vi "MarvinTester.vi"() -> ()   [LabVIEW 2017]
uses:
  <vilib>/Instr/_visa.llb/VISA Configure Serial Port (Instr).vi
panel:
  out "TX":string
  out "RX":string
  out "(hi.lo)":u32 format="%.0x"
  in  "GetOUTIO3":bool
  out "S2 GIO 19":bool
  out "S2 GIO 18":bool
  out "S2 GIO 17":bool
  out "S2 GIO 11":bool
  out "S2 GIO 3":bool
  out "S2 GIO 1":bool
  out "S1 GIO 19":bool
  out "S1 GIO 18":bool
  out "S1 GIO 17":bool
  out "S1 GIO 15":bool
  out "S1 GIO 11":bool
  out "S1 GIO 3":bool
  out "S1 GIO 1":bool
  in  "GetIO 2":bool
  out "S2 GIO 15 R":bool
  in  "Reset":bool
  in  "SetDefault":bool
  out "GetIO":u8[](array[numeric])
  out "Ver":string=" "
  in  "Get  ver":bool
  out "PWM Reading":u32
  out "Time Plot":i32=-1
  out "error out":errorcluster
  in  "stop":bool
  in  "Ring":u16(ring) items=["None", "Moment", "Get IO"]
  out "packet PWM":u8[](array[numeric])
  in  "Tab Control":enum32{"Page 3", "Page 4", "Page 2"}(tab)
  in  "GetIO2":bool
  out "out_io1":u32 format="%.0b"
  in  "SetDAC":bool
  in  "I_O":u32 format="%.0b"
  in  "ADC":bool
  in  "ADC num":u8=3
  out "out_io1 2":u32
  in  "DAC":u32
  out "x*y":dbl
  in  "idx":i32
  in  "TA[idx]":bool
  in  "Disconect 2":bool
  in  "110":bool
  in  "120":bool
  in  "90":bool
  in  "60":bool
  in  "100":bool
  in  "20":bool
  in  "70":bool
  in  "40":bool
  in  "30":bool
  in  "80":bool
  in  "50":bool
  in  "10":bool
  in  "25":bool
  in  "0":bool
  in  "COM Port Marvin":refnum<visa-resource-name>="COM1"
  in  "Connect Marvin":bool
  out "CommIcon Marvin":bool=TRUE
  out "String":string
  in  "K15":bool
  in  "Firmeware":bool
  in  "K16":bool
  in  "K17":bool
  in  "Power":bool
  in  "Fan":bool
  in  "VEnable":bool
  out "CurrSp Graph":cluster{"n":dbl, "T":dbl}[](graph)
  out "Frequency":dbl
  in  "Plot On":bool
  in  "Plot OFF":bool
  in  "Get":bool
  in  "Clear":bool
  in  "Plot Time":i32=70
  out "Load":dbl
  out "String 2":string
  in  "COM Port Control":refnum<visa-resource-name>="COM1"
  in  "Time":i32=-1
  out "err tx":errorcluster
  out "Write array":u8[](array[numeric]) format="%x"
  in  "Flag Stop T":bool
  out "VISA":refnum<visa-resource-name>
  out "CommIcon":bool=TRUE
  out "Read array":u8[](array[numeric]) format="%x"
  out "Cmd Id":u8
  in  "Flag Stop I":bool=TRUE
  out "Int b":i32
  in  "Flag Stop R":bool
  out "TX":bool
  out "RX":bool
  in  "Command Menu 2":u16(ring) items=["Status", "Moment", "Isc threshold", "Vin Vout", "RESET FF", "Open", "Close", "Up Time", "Interval Period", "Nm Of Retries", "On time", "Save Parameters", "Version", "Temperature"]
  out "packet":u8[](array[numeric])
  in  "Isc1":i8
  in  "Add Unit":u8
  in  "Disconect":bool
  in  "Connect":bool
  in  "Stop VI":bool
  out "status":bool
  # "Marvin Tester"
  # "[Hz]"
  # "SW Version"
  # "ver : 00.01.b"
  # "I/O"
  # "ADC"
  # "DAC"
  # "0-4"
  # "V=ADC*3.3/4096"
  # "Term1  -0\nTerm2  -1\nCurr   - 2\nEBAYFAN -3\nTempCPU -4"
  # "b0-Rly1\nb1-Rly2\nb2-Rly3\n....\nb20-Rly20\nb21-Power"
  # "[kHz]"
  # "[N.m]"
  # "[msec]"
  # "ver 0.0.1"
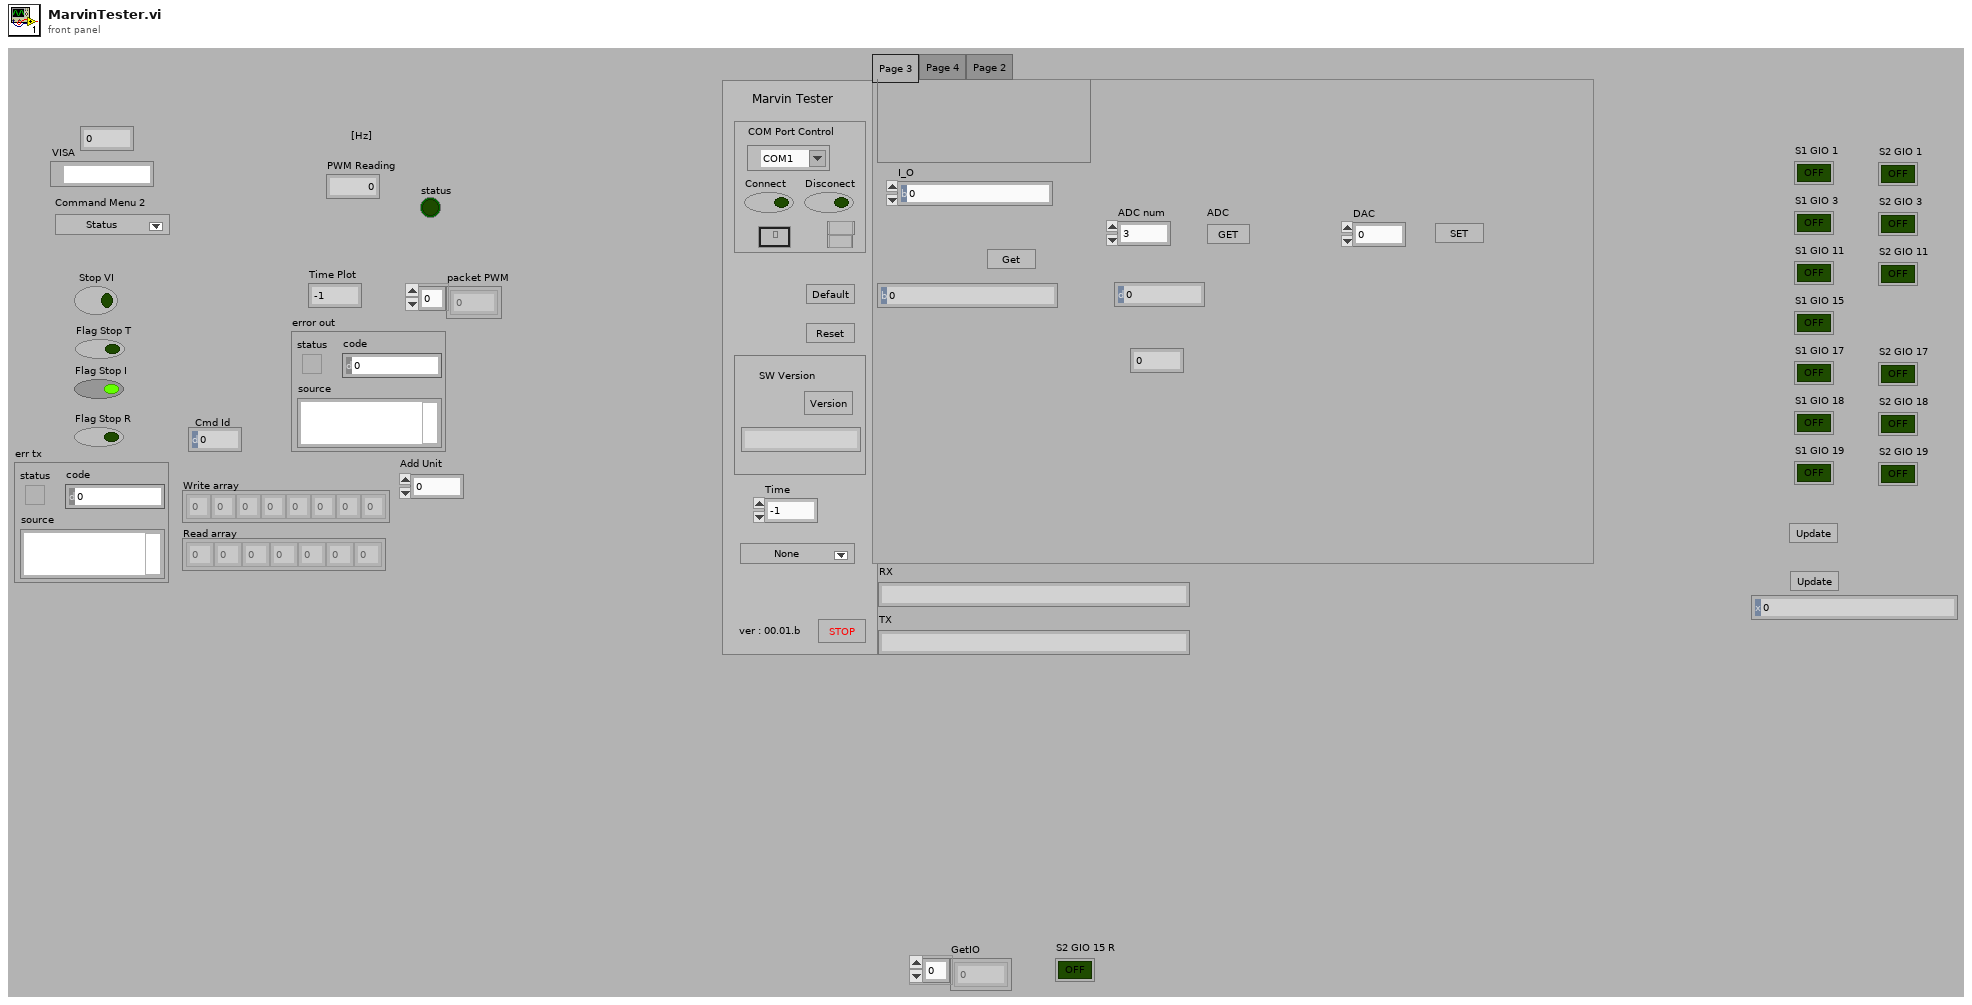
[diagram p1: front panel]
types:
  T1 = cluster{"d1":dbl, "d2":dbl, "d3":dbl, "id":u16, "d4":dbl}
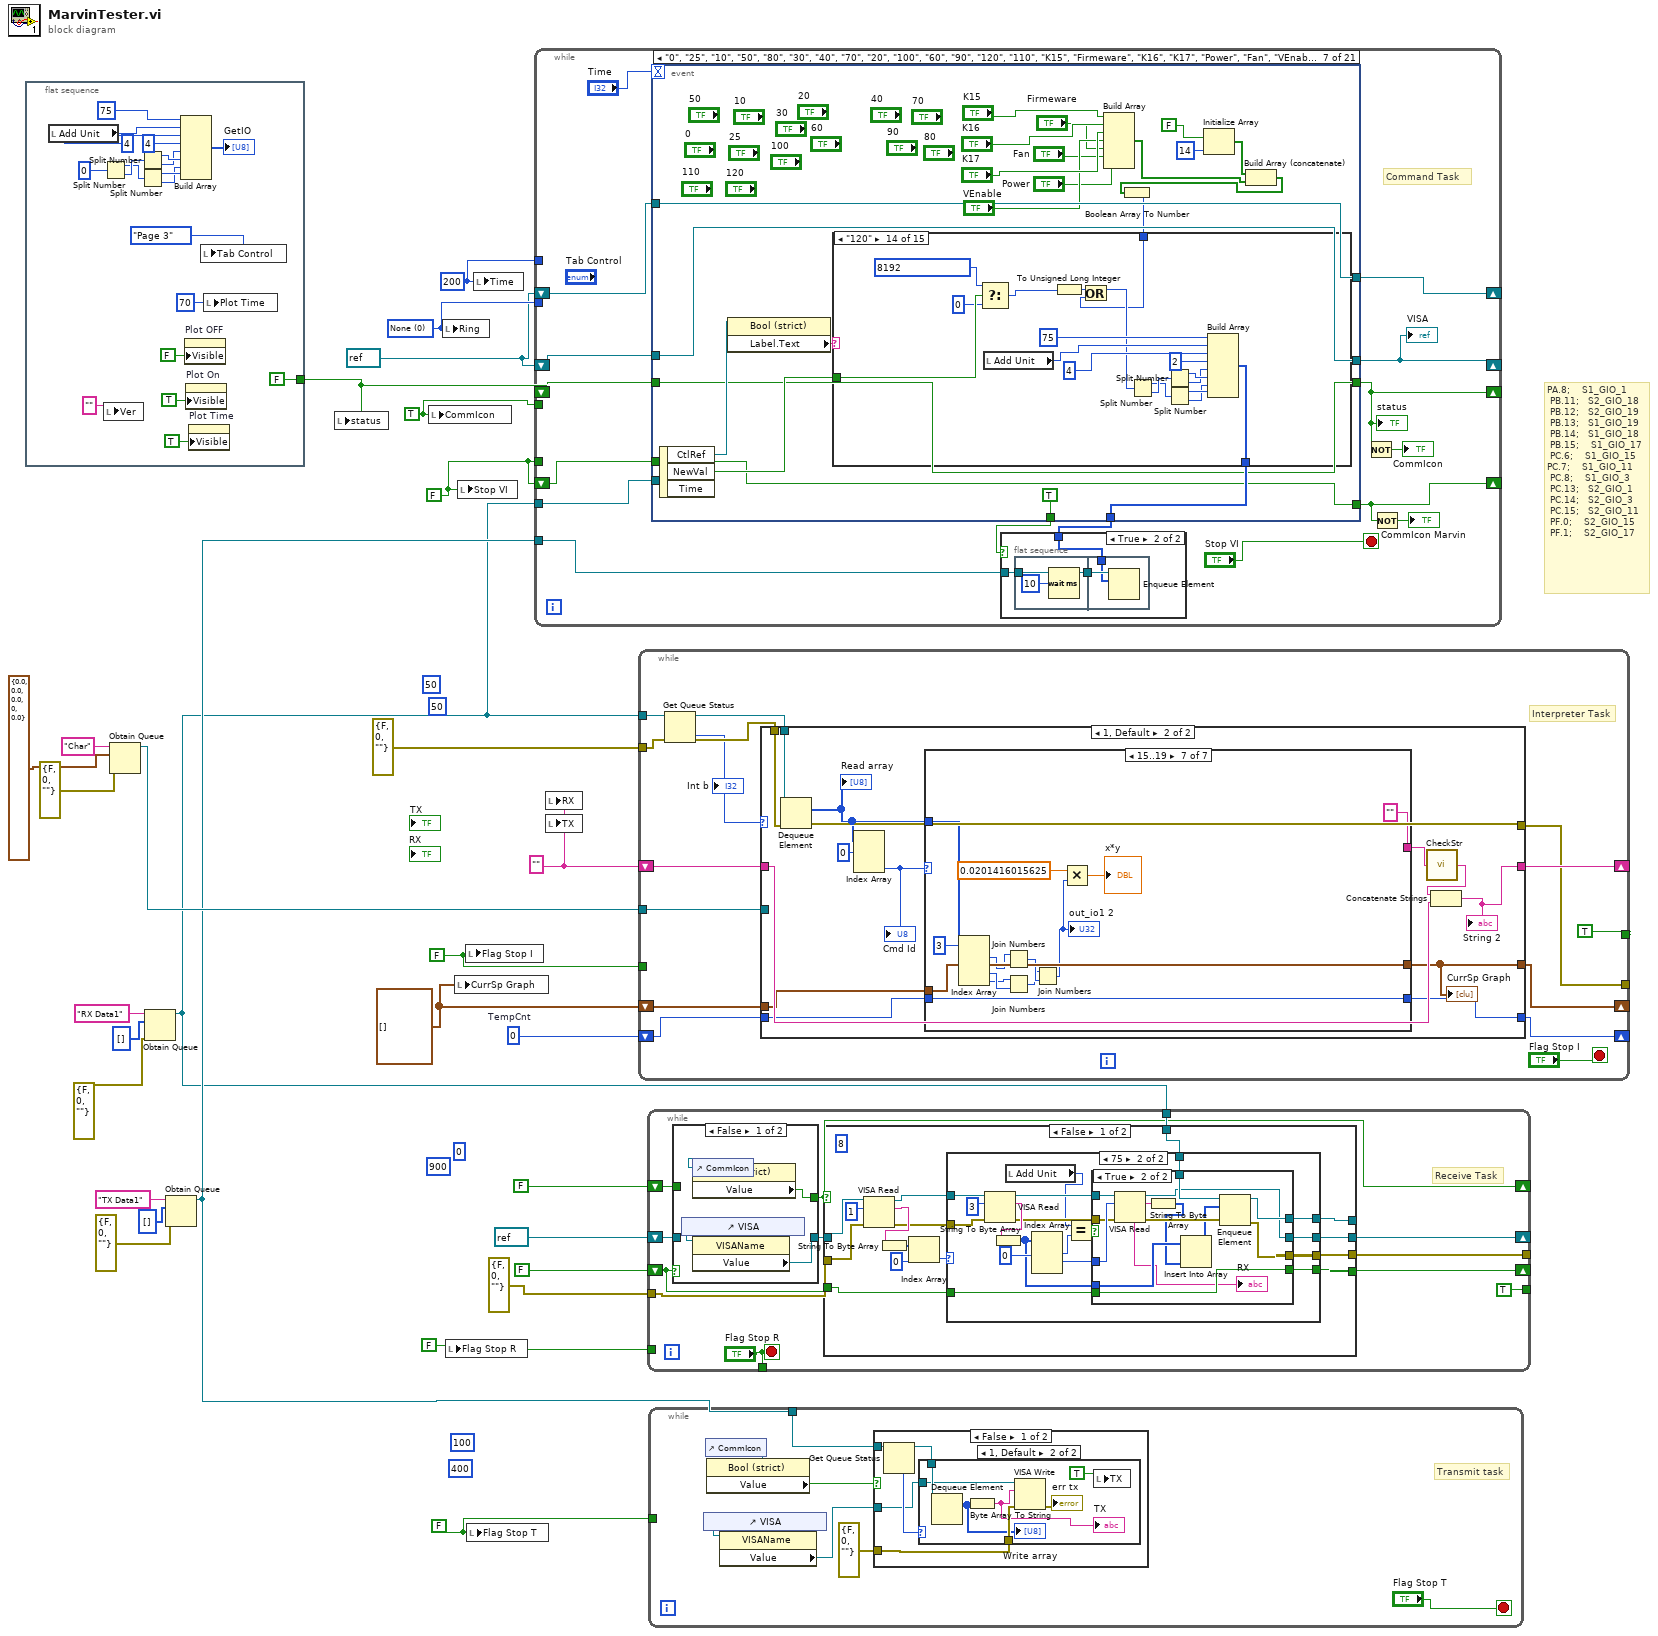
[diagram p0: block diagram]
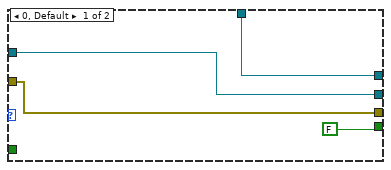
[diagram p3: hidden frame]
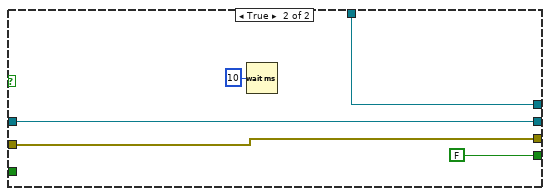
[diagram p5: hidden frame]
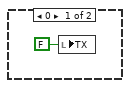
[diagram p6: hidden frame]
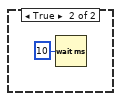
[diagram p7: hidden frame]
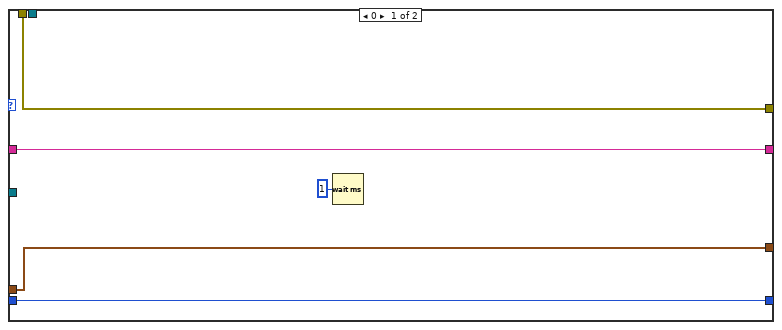
[diagram p8: hidden frame]
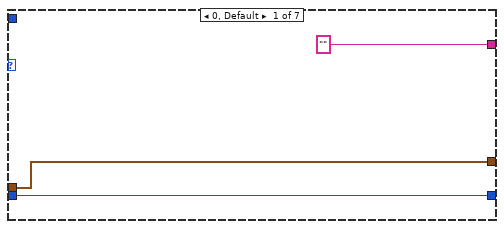
[diagram p9: hidden frame]
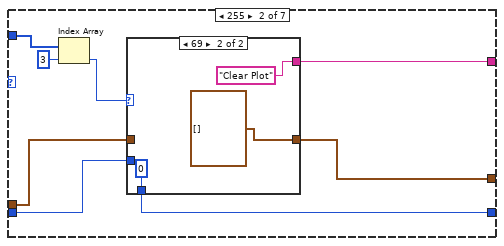
[diagram p10: hidden frame]
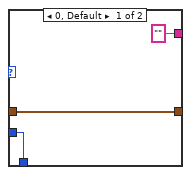
[diagram p11: hidden frame]
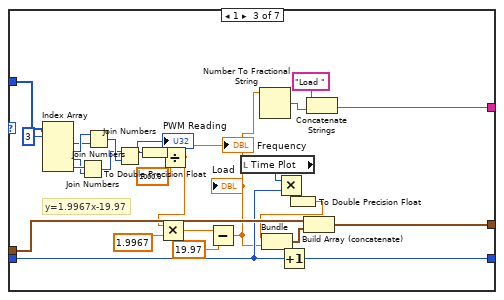
[diagram p12: hidden frame]
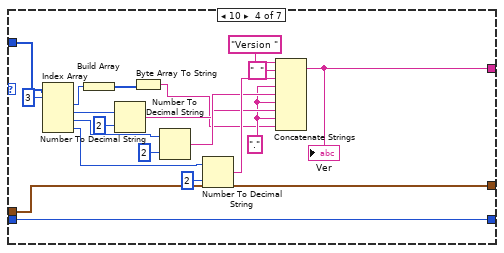
[diagram p13: hidden frame]
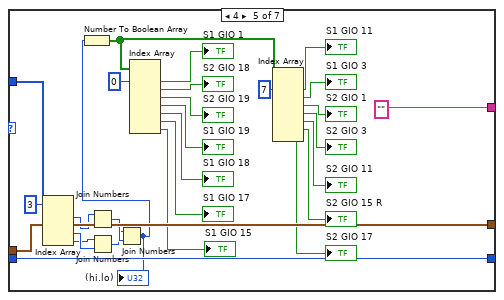
[diagram p14: hidden frame]
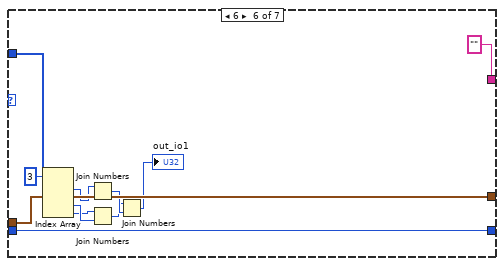
[diagram p15: hidden frame]
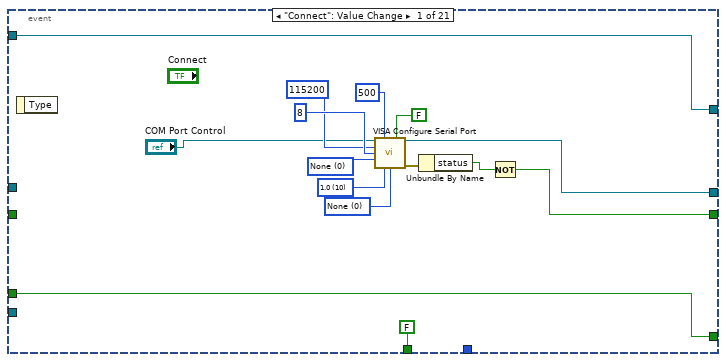
[diagram p17: hidden frame]
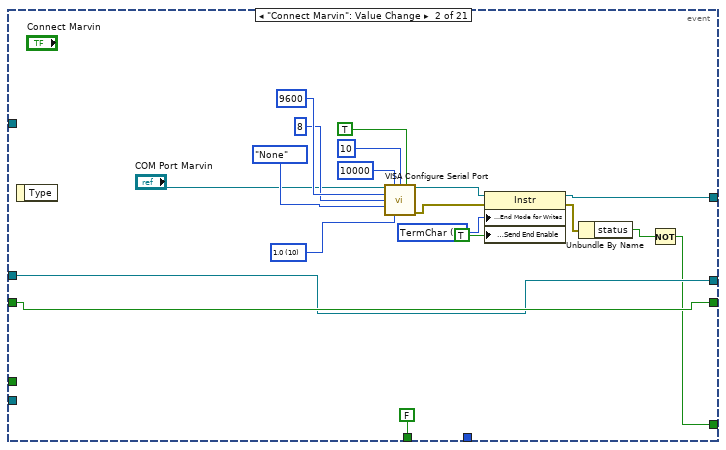
[diagram p18: hidden frame]
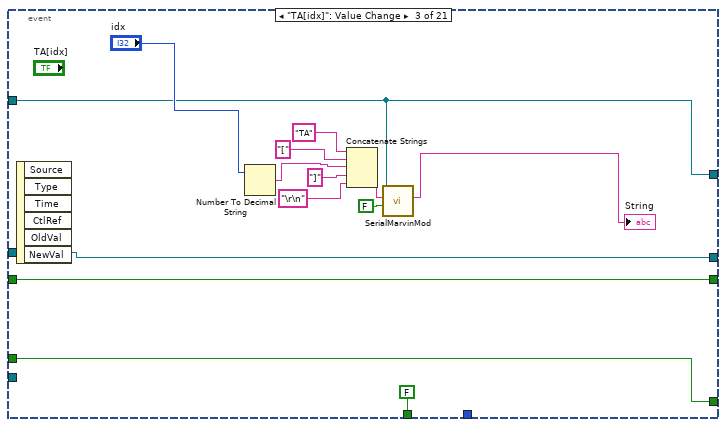
[diagram p19: hidden frame]
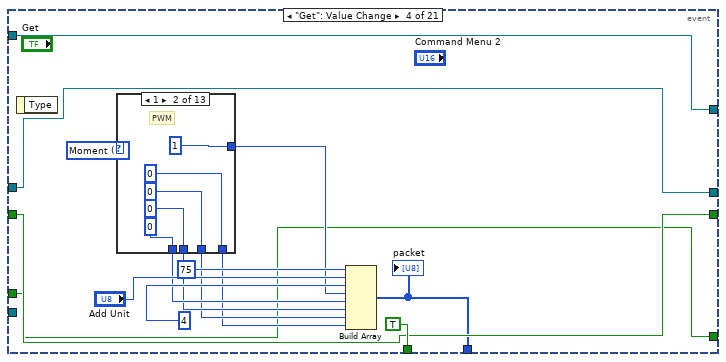
[diagram p20: hidden frame]
diagram:
  w8 = u16 0  # TempCnt
  w5 = cluster{"n":dbl, "T":dbl}[] [] ("Current Graph 4")
  w9 = 200 ("Time")
  w10 = u16 0 items=["None", "Moment"] ("Ring")
  w11 = TRUE ("CommIcon")
  w2 = FALSE
  (unwired) 400 ("Priority")
  (unwired) i64 100 ("Period")
  (unwired) i64 50 ("Period")
  (unwired) 50 ("Priority")
  (unwired) 900 ("Priority")
  (unwired) i64 0 ("Period")
  w14 = FALSE
  w1 = ""
  w28 = FALSE
  w29 = FALSE
  w3 = refnum<visa-resource-name> refnum ("VISA resource name out")
  # "PA.8;   \tS1_GIO_1\n\tPB.11;  \tS2_GIO_18\n\tPB.12;  \tS2_GIO_19\n\tPB.13;  \tS1_GIO_19\n\tPB.14;  \tS1_GIO_18\n\tPB.15;   \tS1_GIO_17\n\tPC.6;   \tS1_GIO_15\nPC.7;   \tS1_GIO_11\n\tPC.8;   \tS1_GIO_3\n\tPC.13;  \tS2_GIO_1\n\tPC.14;  \tS2_GIO_3\n\tPC.15;  \tS2_GIO_11\n\tPF.0;  \t\tS2_GIO_15\n\tPF.1;  \t\tS2_GIO_17"
  n1 = flat-sequence {
    tunnel: [FALSE] -> w7
    frame #0 {
      n2 = local read "Add Unit"() -> (w39:u8)
      n3 = Split Number(x=u32 0) -> (hi(x)=w37:u16, lo(x)=w38:u16)
      n4 = local write "Ver"("" ("Ver")) -> ()
      n5 = Split Number(x=w38) -> (hi(x)=w36:u8, lo(x)=w35:u8)
      n6 = Split Number(x=w37) -> (hi(x)=w34:u8, lo(x)=w33:u8)
      n7 = Build Array(u8 75, w39, u8 4 ("Length"), u8 4, w35, w36, w33, w34) -> (→"GetIO":u8[])
      n8 = property on="Plot OFF" class="Bool"("Visible"=FALSE) -> ()  [unwired: 2 in, 2 out]
      n9 = property on="Plot On" class="Bool"("Visible"=TRUE) -> ()  [unwired: 2 in, 2 out]
      n10 = property on="Plot Time" class="DigNum (strict)"("Visible"=TRUE) -> ()  [unwired: 2 in, 2 out]
      n11 = local write "Tab Control"(enum32{"Page 3", "Page 4", "Page 2"}."Page 3" ("Tab Control")) -> ()
      n12 = local write "Plot Time"(70 ("Plot Time")) -> ()
    }
  }
  n13 = Obtain Queue(name (unnamed)="Char", element data type=T1 {"d1"=0.0, "d2"=0.0, "d3"=0.0, "id"=0, "d4"=0.0}, error in (no error)=errorcluster {"status"=FALSE, "code"=0, "source"=""}) -> (queue out=w19:refnum<queue>)  [unwired: 2 in, 2 out]
  n14 = Obtain Queue(name (unnamed)="RX Data1", element data type=u8[] [], error in (no error)=errorcluster {"status"=FALSE, "code"=0, "source"=""}) -> (queue out=w6:refnum<queue>)  [unwired: 2 in, 2 out]
  n15 = Obtain Queue(name (unnamed)="TX Data1", element data type=u8[] [], error in (no error)=errorcluster {"status"=FALSE, "code"=0, "source"=""}) -> (queue out=w13:refnum<queue>)  [unwired: 2 in, 2 out]
  n16 = local write "status"(w7) -> ()
  n17 = local write "CommIcon"(w11) -> ()
  n18 = local write "Ring"(w10) -> ()
  n19 = local write "Flag Stop R"(w29) -> ()
  n20 = local write "CurrSp Graph"(w5) -> ()
  n21 = local write "Stop VI"(w2) -> ()
  n22 = local write "Flag Stop I"(w28) -> ()
  n23 = local write "Flag Stop T"(w14) -> ()
  n24 = local write "Time"(w9) -> ()
  n25 = while {
    shift-right: [w57] -> _
    shift-left: w3 -> [w64]
    shift-right: [w56] -> _
    shift-left: w7 -> [w63]
    tunnel: w13 -> [w59]
    tunnel: w2 -> [_]
    tunnel: w11 -> [_]
    tunnel: w10 -> [_]
    tunnel: w9 -> [_]
    tunnel: w6 -> [w54]
    shift-right: [w52] -> _
    shift-left: w3 -> [w51]
    shift-right: [w50] -> _
    shift-left: w2 -> [w49]
    stop <- "Stop VI" stop-if-true
    # "Command Task"
    n26 = event shown="[6] \"0\", \"25\", \"10\", \"50\", \"80\", \"30\", \"40\", \"70\", \"20\", \"100\", \"60\", \"90\", \"120\", \"110\", \"K15\", \"Firmeware\", \"K16\", \"K17\", \"Power\", \"Fan\", \"VEnable\": Value Change" {
      selector: _ -> [_ _ _ _ _ _ _ _ _ _ _ _ _ _ _ _ _ _ _ _ _]
      dyn-events: _ -> [_ _ _ _ _ _ _ _ _ _ _ _ _ _ _ _ _ _ _ _ _]
      timeout: "Time" -> [_ _ _ _ _ _ _ _ _ _ _ _ _ _ _ _ _ _ _ _ _]
      tunnel: [w80 w103 w109 w124 w206 w284 w315 w592 w603 w620 w637 w654 w671 w688 w717 w727 w734 w738 refnum<visa-resource-name> refnum ("VISA resource name out") w753 w762] -> w57
      tunnel: w64 -> [_ w103 w109 w124 w206 w284 w315 w592 w603 w620 w637 w654 w671 w688 w717 w727 w734 w738 w749 w753 w762]
      tunnel: [w78 w104 w108 w123 w205 w294 w314 w595 w611 w628 w645 w662 w679 w696 w719 w729 w736 FALSE FALSE w751 w761] -> w56
      tunnel: w63 -> [_ w104 w108 w123 w205 w294 w314 w595 w611 w628 w645 w662 w679 w696 w719 w729 w736 _ _ w751 w761]
      tunnel: [_ _ _ w122 w204 w293 w317 w594 w601 w618 w635 w652 w669 w686 _ _ _ _ _ _ w759] -> w58
      tunnel: [FALSE FALSE FALSE TRUE TRUE TRUE TRUE TRUE TRUE TRUE TRUE TRUE TRUE TRUE FALSE FALSE FALSE FALSE FALSE FALSE w760] -> w60
      tunnel: w54 -> [_ _ _ _ _ _ _ _ _ _ _ _ _ _ _ _ w733 _ _ _ _]
      tunnel: [w73 w90 w110 w121 w201 w282 w313 w587 w600 w617 w634 w651 w668 w685 w702 w721 w731 w739 w745 refnum<visa-resource-name> refnum ("VISA resource name out") w757] -> w52
      tunnel: w51 -> [w73 _ w110 w121 w201 w282 w313 w587 w600 w617 w634 w651 w668 w685 w702 w721 w731 w739 w745 w752 w757]
      tunnel: [w72 w87 w106 w120 w200 w281 w312 w586 w599 w616 w633 w650 w667 w684 w701 w720 w730 w737 w744 FALSE w756] -> w50
      tunnel: w49 -> [w72 _ w106 w120 w200 w281 w312 w586 w599 w616 w633 w650 w667 w684 w701 w720 w730 w737 w744 _ w756]
      event "Connect": Value Change {
        w86 = u16 0 items=["None"=0, "XON/XOFF"=1, "RTS/CTS"=2, "DTR/DSR"=4] ("flow control")
        w85 = u16 10 items=["1.0"=10, "1.5"=15, "2.0"=20] ("stop bits")
        w84 = u16 0 items=["None", "Odd", "Even", "Mark", "Space"] ("parity")
        n27 = event-data() -> ()  [unwired: 1 in, 1 out]
        n28 = call-poly "VISA Configure Serial Port"("VISA resource name"="COM Port Control", "timeout (10sec)"=u32 500, "Enable Termination\nChar (T)"=FALSE ("Enable Termination\nChar (T)"), "baud rate (9600)"=u32 115200 ("baud rate"), "data bits (8)"=u16 8 ("data bits"), "parity (0:none)"=w84, "stop bits (10: 1 bit)"=w85, "flow control (0:none)"=w86) -> ("VISA resource name out"=w80:refnum<visa-resource-name>, "error out"=w77:errorcluster)  [unwired: 6 in]
        n29 = Unbundle By Name(w77) -> ("status"=w79:bool)
        n30 = Not(x=w79) -> (.not. x?=w78:bool)
      }
      event "Connect Marvin": Value Change {
        w102 = u16 2 items=["None", "LastBit", "TermChar", "Break"] ("Serial Settings:Serial End Mode for Writes")
        w95 = u16 10 items=["1.0"=10, "1.5"=15, "2.0"=20] ("stop bits (10: 1 bit)")
        n31 = event-data() -> ()  [unwired: 1 in, 1 out]
        n32 = call-poly "VISA Configure Serial Port"("VISA resource name"="COM Port Marvin", "timeout (10sec)"=u32 10000, "termination char\n(0xA = '\\n' = LF)"=u8 10 ("termination char\n(0xA = '\\n' = LF)"), "Enable Termination\nChar (T)"=TRUE ("Enable Termination\nChar (T)"), "baud rate (9600)"=u32 9600, "data bits (8)"=u16 8, "parity (0:none)"=enum16{"None", "Odd", "Even", "Mark", "Space"}."None", "stop bits (10: 1 bit)"=w95) -> ("VISA resource name out"=w93:refnum<visa-resource-name>, "error out"=w92:errorcluster)  [unwired: 6 in]
        n33 = property class="Instr"(reference=w93, error in=w92, "Serial Settings:End Mode for Writes"=w102, "Message Based Settings:Send End Enable"=TRUE) -> (reference out=w90:refnum<visa-resource-name>, error out=w88:errorcluster)
        n34 = Unbundle By Name(w88) -> ("status"=w89:bool)
        n35 = Not(x=w89) -> (.not. x?=w87:bool)
      }
      event "TA[idx]": Value Change {
        n36 = event-data() -> ()  [unwired: 1 in, 6 out]
        n37 = Number To Decimal String(number="idx") -> (decimal integer string=w113:string)  [unwired: 1 in]
        n38 = Concatenate Strings("TA" ("string"), "[", w113, "]", "\r\n" ("write buffer")) -> (w114:string)
        n39 = call "SerialMarvinMod.vi"("Clear Log"=FALSE, "write buffer"=w114, "VISA resource name"=w110) -> ("read buffer"=→"String":string)  [unwired: 7 in, 1 out]
      }
      event "Get": Value Change {
        w126 = u16 1 items=["Status", "Moment", "Isc threshold", "Vin Vout", "RESET FF", "Open", "Close", "Up Time", "Interval Period", "Nm Of Retries", "On time", "Save Parameters", "Version", "Temperature"] ("Command Menu 3")
        n40 = event-data() -> ()  [unwired: 1 in, 1 out]
        n41 = case shown="1" w126 {
          tunnel: [u8 0 u8 1 u8 2 u8 15 u8 4 u8 4 u8 5 u8 6 u8 7 u8 8 u8 9 u8 10 u8 16] -> w131
          tunnel: [u8 0 u8 0 u8 0 u8 0 u8 0 u8 0 u8 0 u8 0 u8 0 u8 0 u8 0 u8 0 u8 0] -> w129
          tunnel: [u8 0 u8 0 u8 0 u8 0 u8 0 u8 0 u8 0 u8 0 u8 0 u8 0 u8 0 u8 0 u8 0] -> w128
          tunnel: [u8 0 u8 0 "Isc1" u8 0 u8 1 u8 0 u8 0 u8 0 u8 0 u8 0 u8 0 u8 0 u8 0] -> w130
          tunnel: [u8 0 u8 0 u8 0 u8 0 u8 0 u8 0 u8 0 u8 0 u8 0 u8 0 u8 0 u8 0 u8 0] -> w127
          frame 0, Default {
            # "Status"
          }
          frame 1 {
            # "PWM"
          }
          frame 2 {
          }
          frame 3 {
            # "Vout"
          }
          frame 5 {
          }
          frame 6 {
          }
          frame 7 {
          }
          frame 8 {
          }
          frame 9 {
          }
          frame 10 {
          }
          frame 11 {
          }
          frame 12 {
          }
          frame 13 {
          }
        }
        n42 = Build Array(u8 75, "Add Unit", u8 4 ("Length"), w131, w130, w129, w128, w127) -> (w122:u8[])
        "packet" <- w122
      }
      event "Get  ver": Value Change {
        w208 = u16 12 items=["Status", "Moment", "Isc threshold", "Vin Vout", "RESET FF", "Open", "Close", "Up Time", "Interval Period", "Nm Of Retries", "On time", "Save Parameters", "Version", "Temperature"] ("Command Menu 3")
        n43 = event-data() -> ()  [unwired: 1 in, 1 out]
        n44 = local read "Add Unit"() -> (w203:u8)
        n45 = case shown="0, Default" w208 {
          tunnel: [u8 0 u8 1 u8 2 u8 15 u8 4 u8 4 u8 5 u8 6 u8 7 u8 8 u8 9 u8 10 u8 16] -> w213
          tunnel: [u8 0 u8 0 u8 0 u8 0 u8 0 u8 0 u8 0 u8 0 u8 0 u8 0 u8 0 u8 0 u8 0] -> w211
          tunnel: [u8 0 u8 0 u8 0 u8 0 u8 0 u8 0 u8 0 u8 0 u8 0 u8 0 u8 0 u8 0 u8 0] -> w210
          tunnel: [u8 0 u8 0 u8 0 u8 0 u8 1 u8 0 u8 0 u8 0 u8 0 u8 0 u8 0 u8 0 u8 0] -> w212
          tunnel: [u8 0 u8 0 u8 0 u8 0 u8 0 u8 0 u8 0 u8 0 u8 0 u8 0 u8 0 u8 0 u8 0] -> w209
          frame 0, Default {
            # "Status"
          }
          frame 1 {
            # "PWM"
          }
          frame 2 {
          }
          frame 3 {
            # "Vout"
          }
          frame 5 {
          }
          frame 6 {
          }
          frame 7 {
          }
          frame 8 {
          }
          frame 9 {
          }
          frame 10 {
          }
          frame 11 {
          }
          frame 12 {
          }
          frame 13 {
          }
        }
        n46 = local write "Ver"("" ("Ver")) -> ()
        n47 = Build Array(u8 75, w203, u8 4 ("Length"), w213, w212, w211, w210, w209) -> (w204:u8[])
      }
      event "I_O": Value Change {
        n48 = event-data() -> ()  [unwired: 1 in, 3 out]
        n49 = local read "Add Unit"() -> (w292:u8)
        n50 = To Unsigned Long Integer(number="I_O") -> (unsigned 32bit integer=w285:u32)
        n51 = Split Number(x=w285) -> (hi(x)=w290:u16, lo(x)=w291:u16)
        n52 = Split Number(x=w291) -> (hi(x)=w289:u8, lo(x)=w288:u8)
        n53 = Split Number(x=w290) -> (hi(x)=w287:u8, lo(x)=w286:u8)
        n54 = Build Array(u8 75, w292, u8 4 ("Length"), u8 2, w288, w289, w286, w287) -> (w293:u8[])
      }
      event "0", "25", "10", "50", "80", "30", "40", "70", "20", "100", "60", "90", "120", "110", "K15", "Firmeware", "K16", "K17", "Power", "Fan", "VEnable": Value Change {
        n55 = event-data() -> ("CtlRef"=w320:refnum<vi>, "NewVal"=w318:bool)  [unwired: 1 in, 1 out]
        n56 = property class="Bool (strict)"(reference=w320) -> ("Label.Text"=w319:string)  [unwired: 1 in, 2 out]
        n57 = Build Array("K15", "K16", "K17", "VEnable", "Firmeware", "Fan", "Power") -> (w300:bool[])
        n58 = Initialize Array(FALSE, 14 ("dimension size")) -> (w301:bool[])
        n59 = Build Array (concatenate)(w301, w300) -> (w299:bool[])
        n60 = Boolean Array To Number(Boolean array=w299) -> (number=w304:u32)
        n61 = case shown="\"120\"" w319 {
          tunnel: w318 -> [w328 w346 w363 w381 w398 w416 w434 w453 w471 w488 w507 w524 w542 w560 _]
          tunnel: [w325 w343 w360 w378 w395 w413 w431 w450 w468 w485 w504 w521 w539 w557 w573] -> w317
          tunnel: w304 -> [w322 w341 w357 w376 w393 w411 w429 w448 w467 w483 w502 w519 w537 w555 w574]
          frame "0" {
            n62 = Select(t=u32 1 ("number"), s=w328, f=u32 0) -> (s? t:f=w326:u32)
            n63 = local read "Add Unit"() -> (w329:u8)
            n64 = To Unsigned Long Integer(number=w326) -> (unsigned 32bit integer=w323:u32)
            n65 = Or(x=w322, y=w323) -> (x .or. y?=w321:u32)
            n66 = Split Number(x=w321) -> (hi(x)=w334:u16, lo(x)=w335:u16)
            n67 = Split Number(x=w335) -> (hi(x)=w333:u8, lo(x)=w332:u8)
            n68 = Split Number(x=w334) -> (hi(x)=w331:u8, lo(x)=w330:u8)
            n69 = Build Array(u8 75, w329, u8 4 ("Length"), u8 2, w332, w333, w330, w331) -> (w325:u8[])
          }
          frame "10" {
            n70 = Select(t=u32 2 ("number"), s=w346, f=u32 0) -> (s? t:f=w344:u32)
            n71 = local read "Add Unit"() -> (w347:u8)
            n72 = To Unsigned Long Integer(number=w344) -> (unsigned 32bit integer=w340:u32)
            n73 = Or(x=w341, y=w340) -> (x .or. y?=w339:u32)
            n74 = Split Number(x=w339) -> (hi(x)=w352:u16, lo(x)=w353:u16)
            n75 = Split Number(x=w353) -> (hi(x)=w351:u8, lo(x)=w350:u8)
            n76 = Split Number(x=w352) -> (hi(x)=w349:u8, lo(x)=w348:u8)
            n77 = Build Array(u8 75, w347, u8 4 ("Length"), u8 2, w350, w351, w348, w349) -> (w343:u8[])
          }
          frame "20" {
            n78 = Select(t=u32 4 ("number"), s=w363, f=u32 0) -> (s? t:f=w361:u32)
            n79 = local read "Add Unit"() -> (w365:u8)
            n80 = To Unsigned Long Integer(number=w361) -> (unsigned 32bit integer=w359:u32)
            n81 = Or(x=w357, y=w359) -> (x .or. y?=w358:u32)
            n82 = Split Number(x=w358) -> (hi(x)=w370:u16, lo(x)=w371:u16)
            n83 = Split Number(x=w371) -> (hi(x)=w369:u8, lo(x)=w368:u8)
            n84 = Split Number(x=w370) -> (hi(x)=w367:u8, lo(x)=w366:u8)
            n85 = Build Array(u8 75, w365, u8 4 ("Length"), u8 2, w368, w369, w366, w367) -> (w360:u8[])
          }
          frame "25" {
            n86 = Select(t=u32 8 ("number"), s=w381, f=u32 0) -> (s? t:f=w379:u32)
            n87 = local read "Add Unit"() -> (w383:u8)
            n88 = To Unsigned Long Integer(number=w379) -> (unsigned 32bit integer=w377:u32)
            n89 = Or(x=w376, y=w377) -> (x .or. y?=w375:u32)
            n90 = Split Number(x=w375) -> (hi(x)=w388:u16, lo(x)=w389:u16)
            n91 = Split Number(x=w389) -> (hi(x)=w387:u8, lo(x)=w386:u8)
            n92 = Split Number(x=w388) -> (hi(x)=w385:u8, lo(x)=w384:u8)
            n93 = Build Array(u8 75, w383, u8 4 ("Length"), u8 2, w386, w387, w384, w385) -> (w378:u8[])
          }
          frame "30" {
            n94 = Select(t=u32 16 ("number"), s=w398, f=u32 0) -> (s? t:f=w396:u32)
            n95 = local read "Add Unit"() -> (w400:u8)
            n96 = To Unsigned Long Integer(number=w396) -> (unsigned 32bit integer=w401:u32)
            n97 = Or(x=w401, y=w393) -> (x .or. y?=w394:u32)
            n98 = Split Number(x=w394) -> (hi(x)=w406:u16, lo(x)=w407:u16)
            n99 = Split Number(x=w407) -> (hi(x)=w405:u8, lo(x)=w404:u8)
            n100 = Split Number(x=w406) -> (hi(x)=w403:u8, lo(x)=w402:u8)
            n101 = Build Array(u8 75, w400, u8 4 ("Length"), u8 2, w404, w405, w402, w403) -> (w395:u8[])
          }
          frame "40" {
            n102 = Select(t=u32 32 ("number"), s=w416, f=u32 0) -> (s? t:f=w414:u32)
            n103 = local read "Add Unit"() -> (w418:u8)
            n104 = To Unsigned Long Integer(number=w414) -> (unsigned 32bit integer=w419:u32)
            n105 = Or(x=w411, y=w419) -> (x .or. y?=w412:u32)
            n106 = Split Number(x=w412) -> (hi(x)=w424:u16, lo(x)=w425:u16)
            n107 = Split Number(x=w425) -> (hi(x)=w423:u8, lo(x)=w422:u8)
            n108 = Split Number(x=w424) -> (hi(x)=w421:u8, lo(x)=w420:u8)
            n109 = Build Array(u8 75, w418, u8 4 ("Length"), u8 2, w422, w423, w420, w421) -> (w413:u8[])
          }
          frame "50" {
            n110 = Select(t=u32 64 ("number"), s=w434, f=u32 0) -> (s? t:f=w432:u32)
            n111 = local read "Add Unit"() -> (w436:u8)
            n112 = To Unsigned Long Integer(number=w432) -> (unsigned 32bit integer=w437:u32)
            n113 = Or(x=w429, y=w437) -> (x .or. y?=w430:u32)
            n114 = Split Number(x=w430) -> (hi(x)=w442:u16, lo(x)=w443:u16)
            n115 = Split Number(x=w443) -> (hi(x)=w441:u8, lo(x)=w440:u8)
            n116 = Split Number(x=w442) -> (hi(x)=w439:u8, lo(x)=w438:u8)
            n117 = Build Array(u8 75, w436, u8 4 ("Length"), u8 2, w440, w441, w438, w439) -> (w431:u8[])
          }
          frame "60" {
            n118 = Select(t=u32 128 ("number"), s=w453, f=u32 0) -> (s? t:f=w451:u32)
            n119 = local read "Add Unit"() -> (w455:u8)
            n120 = To Unsigned Long Integer(number=w451) -> (unsigned 32bit integer=w449:u32)
            n121 = Or(x=w448, y=w449) -> (x .or. y?=w447:u32)
            n122 = Split Number(x=w447) -> (hi(x)=w460:u16, lo(x)=w461:u16)
            n123 = Split Number(x=w461) -> (hi(x)=w459:u8, lo(x)=w458:u8)
            n124 = Split Number(x=w460) -> (hi(x)=w457:u8, lo(x)=w456:u8)
            n125 = Build Array(u8 75, w455, u8 4 ("Length"), u8 2, w458, w459, w456, w457) -> (w450:u8[])
          }
          frame "70" {
            n126 = Select(t=u32 256 ("number"), s=w471, f=u32 0) -> (s? t:f=w469:u32)
            n127 = local read "Add Unit"() -> (w473:u8)
            n128 = To Unsigned Long Integer(number=w469) -> (unsigned 32bit integer=w466:u32)
            n129 = Or(x=w467, y=w466) -> (x .or. y?=w465:u32)
            n130 = Split Number(x=w465) -> (hi(x)=w478:u16, lo(x)=w479:u16)
            n131 = Split Number(x=w479) -> (hi(x)=w477:u8, lo(x)=w476:u8)
            n132 = Split Number(x=w478) -> (hi(x)=w475:u8, lo(x)=w474:u8)
            n133 = Build Array(u8 75, w473, u8 4 ("Length"), u8 2, w476, w477, w474, w475) -> (w468:u8[])
          }
          frame "80" {
            n134 = Select(t=u32 512 ("number"), s=w488, f=u32 0) -> (s? t:f=w486:u32)
            n135 = local read "Add Unit"() -> (w490:u8)
            n136 = To Unsigned Long Integer(number=w486) -> (unsigned 32bit integer=w491:u32)
            n137 = Or(x=w483, y=w491) -> (x .or. y?=w484:u32)
            n138 = Split Number(x=w484) -> (hi(x)=w496:u16, lo(x)=w497:u16)
            n139 = Split Number(x=w497) -> (hi(x)=w495:u8, lo(x)=w494:u8)
            n140 = Split Number(x=w496) -> (hi(x)=w493:u8, lo(x)=w492:u8)
            n141 = Build Array(u8 75, w490, u8 4 ("Length"), u8 2, w494, w495, w492, w493) -> (w485:u8[])
          }
          frame "90" {
            n142 = Select(t=u32 1024 ("number"), s=w507, f=u32 0) -> (s? t:f=w505:u32)
            n143 = local read "Add Unit"() -> (w509:u8)
            n144 = To Unsigned Long Integer(number=w505) -> (unsigned 32bit integer=w503:u32)
            n145 = Or(x=w502, y=w503) -> (x .or. y?=w501:u32)
            n146 = Split Number(x=w501) -> (hi(x)=w514:u16, lo(x)=w515:u16)
            n147 = Split Number(x=w515) -> (hi(x)=w513:u8, lo(x)=w512:u8)
            n148 = Split Number(x=w514) -> (hi(x)=w511:u8, lo(x)=w510:u8)
            n149 = Build Array(u8 75, w509, u8 4 ("Length"), u8 2, w512, w513, w510, w511) -> (w504:u8[])
          }
          frame "100" {
            n150 = Select(t=u32 2048 ("number"), s=w524, f=u32 0) -> (s? t:f=w522:u32)
            n151 = local read "Add Unit"() -> (w526:u8)
            n152 = To Unsigned Long Integer(number=w522) -> (unsigned 32bit integer=w527:u32)
            n153 = Or(x=w519, y=w527) -> (x .or. y?=w520:u32)
            n154 = Split Number(x=w520) -> (hi(x)=w532:u16, lo(x)=w533:u16)
            n155 = Split Number(x=w533) -> (hi(x)=w531:u8, lo(x)=w530:u8)
            n156 = Split Number(x=w532) -> (hi(x)=w529:u8, lo(x)=w528:u8)
            n157 = Build Array(u8 75, w526, u8 4 ("Length"), u8 2, w530, w531, w528, w529) -> (w521:u8[])
          }
          frame "110" {
            n158 = local read "Add Unit"() -> (w544:u8)
            n159 = Select(t=u32 4096 ("number"), s=w542, f=u32 0) -> (s? t:f=w540:u32)
            n160 = To Unsigned Long Integer(number=w540) -> (unsigned 32bit integer=w545:u32)
            n161 = Or(x=w537, y=w545) -> (x .or. y?=w538:u32)
            n162 = Split Number(x=w538) -> (hi(x)=w550:u16, lo(x)=w551:u16)
            n163 = Split Number(x=w551) -> (hi(x)=w549:u8, lo(x)=w548:u8)
            n164 = Split Number(x=w550) -> (hi(x)=w547:u8, lo(x)=w546:u8)
            n165 = Build Array(u8 75, w544, u8 4 ("Length"), u8 2, w548, w549, w546, w547) -> (w539:u8[])
          }
          frame "120" {
            n166 = Select(t=u32 8192 ("number"), s=w560, f=u32 0) -> (s? t:f=w558:u32)
            n167 = local read "Add Unit"() -> (w562:u8)
            n168 = To Unsigned Long Integer(number=w558) -> (unsigned 32bit integer=w563:u32)
            n169 = Or(x=w563, y=w555) -> (x .or. y?=w556:u32)
            n170 = Split Number(x=w556) -> (hi(x)=w568:u16, lo(x)=w569:u16)
            n171 = Split Number(x=w569) -> (hi(x)=w567:u8, lo(x)=w566:u8)
            n172 = Split Number(x=w568) -> (hi(x)=w565:u8, lo(x)=w564:u8)
            n173 = Build Array(u8 75, w562, u8 4 ("Length"), u8 2, w566, w567, w564, w565) -> (w557:u8[])
          }
          frame Default {
            n174 = local read "Add Unit"() -> (w575:u8)
            n175 = To Unsigned Long Integer(number=w574) -> (unsigned 32bit integer=w576:u32)
            n176 = Split Number(x=w576) -> (hi(x)=w581:u16, lo(x)=w582:u16)
            n177 = Split Number(x=w582) -> (hi(x)=w580:u8, lo(x)=w579:u8)
            n178 = Split Number(x=w581) -> (hi(x)=w578:u8, lo(x)=w577:u8)
            n179 = Build Array(u8 75, w575, u8 4 ("Length"), u8 2, w579, w580, w577, w578) -> (w573:u8[])
          }
        }
      }
      event "ADC": Value Change {
        w588 = u8 0 ("element")
        n180 = event-data() -> ()  [unwired: 1 in, 3 out]
        n181 = local read "Add Unit"() -> (w593:u8)
        n182 = Add(x="ADC num", y=u8 15) -> (x+y=w590:u8)
        n183 = Build Array(u8 75, w593, u8 4 ("Length"), w590, w588, w588, w588, w588) -> (w594:u8[])
      }
      event "GetIO 2": Value Change {
        n184 = event-data() -> ()  [unwired: 1 in, 1 out]
        n185 = local read "Add Unit"() -> (w610:u8)
        n186 = Split Number(x=u32 0) -> (hi(x)=w608:u16, lo(x)=w609:u16)
        n187 = Split Number(x=w609) -> (hi(x)=w607:u8, lo(x)=w606:u8)
        n188 = Split Number(x=w608) -> (hi(x)=w605:u8, lo(x)=w604:u8)
        n189 = Build Array(u8 75, w610, u8 4 ("Length"), u8 4, w606, w607, w604, w605) -> (w601:u8[])
        n190 = local write "GetIO"(w601) -> ()
      }
      event "SetDefault": Value Change {
        n191 = event-data() -> ()  [unwired: 1 in, 1 out]
        n192 = local read "Add Unit"() -> (w627:u8)
        n193 = Split Number(x=u32 0) -> (hi(x)=w625:u16, lo(x)=w626:u16)
        n194 = Split Number(x=w626) -> (hi(x)=w624:u8, lo(x)=w623:u8)
        n195 = Split Number(x=w625) -> (hi(x)=w622:u8, lo(x)=w621:u8)
        n196 = Build Array(u8 75, w627, u8 4 ("Length"), u8 9, w623, w624, w621, w622) -> (w618:u8[])
        n197 = local write "GetIO"(w618) -> ()
      }
      event "Reset": Value Change {
        n198 = event-data() -> ()  [unwired: 1 in, 1 out]
        n199 = local read "Add Unit"() -> (w644:u8)
        n200 = Split Number(x=u32 0) -> (hi(x)=w642:u16, lo(x)=w643:u16)
        n201 = Split Number(x=w643) -> (hi(x)=w641:u8, lo(x)=w640:u8)
        n202 = Split Number(x=w642) -> (hi(x)=w639:u8, lo(x)=w638:u8)
        n203 = Build Array(u8 75, w644, u8 4 ("Length"), u8 11, w640, w641, w638, w639) -> (w635:u8[])
        n204 = local write "GetIO"(w635) -> ()
      }
      event "GetIO2": Value Change {
        n205 = event-data() -> ()  [unwired: 1 in, 1 out]
        n206 = local read "Add Unit"() -> (w661:u8)
        n207 = Split Number(x=u32 0) -> (hi(x)=w659:u16, lo(x)=w660:u16)
        n208 = Split Number(x=w660) -> (hi(x)=w658:u8, lo(x)=w657:u8)
        n209 = Split Number(x=w659) -> (hi(x)=w656:u8, lo(x)=w655:u8)
        n210 = Build Array(u8 75, w661, u8 4 ("Length"), u8 6, w657, w658, w655, w656) -> (w652:u8[])
      }
      event "SetDAC": Value Change {
        n211 = event-data() -> ()  [unwired: 1 in, 1 out]
        n212 = local read "Add Unit"() -> (w678:u8)
        n213 = Split Number(x="DAC") -> (hi(x)=w676:u16, lo(x)=w677:u16)
        n214 = Split Number(x=w677) -> (hi(x)=w675:u8, lo(x)=w674:u8)
        n215 = Split Number(x=w676) -> (hi(x)=w673:u8, lo(x)=w672:u8)
        n216 = Build Array(u8 75, w678, u8 4 ("Length"), u8 7, w674, w675, w672, w673) -> (w669:u8[])
      }
      event "GetOUTIO3": Value Change {
        n217 = event-data() -> ()  [unwired: 1 in, 1 out]
        n218 = local read "Add Unit"() -> (w695:u8)
        n219 = Split Number(x=u32 0) -> (hi(x)=w693:u16, lo(x)=w694:u16)
        n220 = Split Number(x=w694) -> (hi(x)=w692:u8, lo(x)=w691:u8)
        n221 = Split Number(x=w693) -> (hi(x)=w690:u8, lo(x)=w689:u8)
        n222 = Build Array(u8 75, w695, u8 4 ("Length"), u8 8, w691, w692, w689, w690) -> (w686:u8[])
      }
      event "Plot On": Value Change {
        w707 = u16 1 items=["None", "Moment"] ("Ring")
        n223 = event-data() -> ()  [unwired: 1 in, 1 out]
        n224 = local read "Add Unit"() -> (w716:u8)
        n225 = local write "Ring"(w707) -> ()
        n226 = Build Array(u8 75, w716, u8 4 ("Length"), u8 1, u8 0, u8 0, u8 0, u8 0) -> (→"packet PWM":u8[])
        n227 = local write "Time"("Plot Time") -> ()
        n228 = property on="Plot OFF" class="Bool"("Visible"=TRUE) -> ()  [unwired: 2 in, 2 out]
        n229 = property on="Plot On" class="Bool"("Visible"=FALSE) -> ()  [unwired: 2 in, 2 out]
        n230 = property on="Plot Time" class="DigNum (strict)"("Visible"=FALSE) -> ()  [unwired: 2 in, 2 out]
        "Time Plot" <- "Plot Time"
      }
      event "Plot OFF": Value Change {
        w726 = u16 0 items=["None", "Moment"] ("Ring")
        n231 = event-data() -> ()  [unwired: 1 in, 5 out]
        n232 = local write "Time"(200 ("Time")) -> ()
        n233 = local write "Ring"(w726) -> ()
        n234 = property on="Plot Time" class="DigNum (strict)"("Visible"=TRUE) -> ()  [unwired: 2 in, 2 out]
        n235 = property on="Plot OFF" class="Bool"("Visible"=FALSE) -> ()  [unwired: 2 in, 2 out]
        n236 = property on="Plot On" class="Bool"("Visible"=TRUE) -> ()  [unwired: 2 in, 2 out]
      }
      event "Clear": Value Change {
        n237 = event-data() -> ()  [unwired: 1 in, 5 out]
        n238 = Enqueue Element(queue=w733, element=u8[] [0, 0, 255, 69]) -> ()  [unwired: 1 in, 4 out]
      }
      event "stop": Value Change {
        w740 = TRUE ("Flag Stop R")
        n239 = event-data() -> ()  [unwired: 1 in, 5 out]
        n240 = VISA Close(VISA resource name=w738) -> (error out=→"error out":errorcluster)  [unwired: 1 in]
        n241 = local write "Flag Stop T"(w740) -> ()
        n242 = local write "Flag Stop R"(w740) -> ()
        n243 = local write "Flag Stop I"(w740) -> ()
        n244 = local write "Stop VI"(w740) -> ()
      }
      event "Disconect": Value Change {
        n245 = event-data() -> ()  [unwired: 1 in, 5 out]
        n246 = VISA Close(VISA resource name=w749) -> ()  [unwired: 1 in, 1 out]
      }
      event "Disconect 2": Value Change {
        n247 = event-data() -> ()  [unwired: 1 in, 5 out]
        n248 = VISA Close(VISA resource name=w752) -> ()  [unwired: 1 in, 1 out]
      }
      event Timeout {
        n249 = event-data() -> ()  [unwired: 1 in, 1 out]
        n250 = case shown="0, Default" "Ring" {
          tunnel: [FALSE TRUE TRUE] -> w760
          tunnel: [u8[] [] ("packet PWM") w765 w767] -> w759
          frame 0, Default {
          }
          frame 1 {
            n251 = local read "packet PWM"() -> (w765:u8[])
          }
          frame 2 {
            n252 = local read "GetIO"() -> (w767:u8[])
          }
        }
      }
    }
    "status" <- w56
    "VISA" <- w57
    n253 = case shown="True" w60 {
      tunnel: w59 -> [_ w67]
      tunnel: w58 -> [_ w66]
      frame False {
      }
      frame True {
        n254 = flat-sequence {
          tunnel: w67 -> [w69]
          tunnel: [w69] -> w65
          tunnel: w66 -> [w70]
          tunnel: w65 -> [w71]
          frame #0 {
            n255 = Wait (ms)(milliseconds to wait=u32 10) -> ()  [unwired: 1 out]
          }
          frame #1 {
            n256 = Enqueue Element(queue=w71, element=w70) -> ()  [unwired: 1 in, 4 out]
          }
        }
      }
    }
    n257 = Not(x=w56) -> (.not. x?=→"CommIcon":bool)
    n258 = Not(x=w50) -> (.not. x?=→"CommIcon Marvin":bool)
  }
  n259 = local write "RX"(w1) -> ()
  n260 = local write "TX"(w1) -> ()
  n261 = while {
    tunnel: w6 -> [w783]
    tunnel: errorcluster {"status"=FALSE, "code"=0, "source"=""} ("error out") -> [w782]
    tunnel: [w773] -> _
    tunnel: w28 -> [_]
    tunnel: [TRUE] -> _
    shift-right: [w778] -> _
    shift-left: w1 -> [w777]
    tunnel: w19 -> [w775]
    shift-right: [w769] -> _
    shift-left: w5 -> [w772]
    shift-right: [w770] -> _
    shift-left: w8 -> [w771]
    stop <- "Flag Stop I" stop-if-true
    # "Interpreter Task"
    n262 = Get Queue Status(queue=w783, error in (no error)=w782) -> (queue out=w781:refnum<queue>, error out=w776:errorcluster, # elements in queue=w774:i32)  [unwired: 6 out]
    "Int b" <- w774
    n263 = case shown="1, Default" w774 {
      tunnel: w781 -> [_ w802]
      tunnel: w776 -> [w788 w800]
      tunnel: [w788 w801] -> w773
      tunnel: [w787 w797] -> w778
      tunnel: w777 -> [w787 w799]
      tunnel: w775 -> [_ _]
      tunnel: w772 -> [w786 w792]
      tunnel: [w786 w789] -> w769
      tunnel: w771 -> [w785 w791]
      tunnel: [w785 w790] -> w770
      frame 0 {
        n264 = Wait (ms)(milliseconds to wait=u32 1) -> ()  [unwired: 1 out]
      }
      frame 1, Default {
        n265 = Dequeue Element(queue=w802, error in (no error)=w800) -> (element=w798:u8[], error out=w801:errorcluster)  [unwired: 3 out]
        "Read array" <- w798
        n266 = Index Array(array=w798, index #1=0 ("index")) -> (element #3=w794:u8)  [unwired: 2 in, 2 out]
        "Cmd Id" <- w794
        n267 = case shown="15..19" w794 {
          tunnel: w798 -> [_ w813 w838 w862 w892 w904 w918]
          tunnel: ["" w810 w837 w849 "" "" ""] -> w793
          tunnel: w792 -> [w804 w809 w832 w864 w894 w906 w920]
          tunnel: [w804 w808 w831 w864 w894 w906 w920] -> w789
          tunnel: w791 -> [w803 w807 w830 w863 w893 w905 w919]
          tunnel: [w803 w806 w827 w863 w893 w905 w919] -> w790
          frame 0, Default {
          }
          frame 255 {
            n268 = Index Array(array=w813, index=3) -> (element=w811:u8)
            n269 = case shown="69" w811 {
              tunnel: ["" "Clear Plot"] -> w810
              tunnel: [w816 cluster{"n":dbl, "T":dbl}[] [] ("Current Graph 4")] -> w808
              tunnel: w809 -> [w816 _]
              tunnel: w807 -> [w814 _]
              tunnel: [w814 u16 0 ("TempCnt")] -> w806
              frame 0, Default {
              }
              frame 69 {
              }
            }
          }
          frame 1 {
            # "y=1.9967x-19.97"
            n270 = Index Array(array=w838, index #1=3 ("index")) -> (element #1=w841:u8, element #2=w843:u8, element #3=w844:u8, element #4=w845:u8)  [unwired: 3 in]
            n271 = Join Numbers(hi=w845, lo=w844) -> ((hi.lo)=w839:u16)
            n272 = Join Numbers(hi=w843, lo=w841) -> ((hi.lo)=w840:u16)
            n273 = Join Numbers(hi=w839, lo=w840) -> ((hi.lo)=w836:u32)
            "PWM Reading" <- w836
            n274 = To Double Precision Float(number=w836) -> (double precision float=w835:dbl)
            n275 = Divide(x=w835, y=1000.0) -> (x/y=w824:dbl)
            "Frequency" <- w824
            n276 = Multiply(x=w824, y=1.9967) -> (x*y=w823:dbl)
            n277 = Subtract(x=w823, y=19.97) -> (x-y=w820:dbl)
            "Load" <- w820
            n278 = local read "Time Plot"() -> (w826:i32)
            n279 = Number To Fractional String(number=w820) -> (F-format string=w821:string)  [unwired: 3 in]
            n280 = Multiply(x=w826, y=w830) -> (x*y=w829:i32)
            n281 = Increment(x=w830) -> (x+1=w827:u16)
            n282 = To Double Precision Float(number=w829) -> (double precision float=w828:dbl)
            n283 = Bundle(w828, w820) -> (w833:cluster{dbl, dbl})  [unwired: 1 in]
            n284 = Build Array (concatenate)(w832, w833) -> (w831:cluster{"n":dbl, "T":dbl}[])
            n285 = Concatenate Strings("Load ", w821) -> (w837:string)
          }
          frame 10 {
            w848 = "." ("string")
            n286 = Index Array(array=w862, index #1=3 ("index")) -> (element #1=w858:u8, element #2=w861:u8, element #3=w860:u8, element #4=w859:u8)  [unwired: 3 in]
            n287 = Build Array(w858) -> (w857:u8[])
            n288 = Number To Decimal String(number=w861, width (-)=i16 2) -> (decimal integer string=w853:string)
            n289 = Byte Array To String(unsigned byte array=w857) -> (string=w847:string)
            n290 = Number To Decimal String(number=w860, width (-)=i16 2) -> (decimal integer string=w854:string)
            n291 = Number To Decimal String(number=w859, width (-)=i16 2) -> (decimal integer string=w856:string)
            n292 = Concatenate Strings("Version ", "  " ("string"), w856, w848, w854, w848, w853, w848, w847) -> (w849:string)
            "Ver" <- w849
          }
          frame 4 {
            n293 = Index Array(array=w892, index #1=3 ("index")) -> (element #1=w890:u8, element #2=w889:u8, element #3=w888:u8, element #4=w887:u8)  [unwired: 3 in]
            n294 = Join Numbers(hi=w889, lo=w890) -> ((hi.lo)=w886:u16)
            n295 = Join Numbers(hi=w887, lo=w888) -> ((hi.lo)=w885:u16)
            n296 = Join Numbers(hi=w885, lo=w886) -> ((hi.lo)=w884:u32)
            "(hi.lo)" <- w884
            n297 = Number To Boolean Array(number=w884) -> (Boolean array=w874:bool[])
            n298 = Index Array(array=w874, index #1=0 ("index")) -> (element #1=→"S1 GIO 1":bool, element #2=→"S2 GIO 18":bool, element #3=→"S2 GIO 19":bool, element #4=→"S1 GIO 19":bool, element #5=→"S1 GIO 18":bool, element #6=→"S1 GIO 17":bool, element #7=→"S1 GIO 15":bool)  [unwired: 6 in]
            n299 = Index Array(array=w874, index #1=7 ("index")) -> (element #1=→"S1 GIO 11":bool, element #2=→"S1 GIO 3":bool, element #3=→"S2 GIO 1":bool, element #4=→"S2 GIO 3":bool, element #5=→"S2 GIO 11":bool, element #6=→"S2 GIO 15 R":bool, element #7=→"S2 GIO 17":bool)  [unwired: 6 in]
          }
          frame 6 {
            n300 = Index Array(array=w904, index #1=3 ("index")) -> (element #1=w902:u8, element #2=w901:u8, element #3=w900:u8, element #4=w899:u8)  [unwired: 3 in]
            n301 = Join Numbers(hi=w901, lo=w902) -> ((hi.lo)=w898:u16)
            n302 = Join Numbers(hi=w899, lo=w900) -> ((hi.lo)=w897:u16)
            n303 = Join Numbers(hi=w897, lo=w898) -> ((hi.lo)=→"out_io1":u32)
          }
          frame 15..19 {
            n304 = Index Array(array=w918, index #1=3 ("index")) -> (element #1=w916:u8, element #2=w915:u8, element #3=w914:u8, element #4=w913:u8)  [unwired: 3 in]
            n305 = Join Numbers(hi=w915, lo=w916) -> ((hi.lo)=w912:u16)
            n306 = Join Numbers(hi=w913, lo=w914) -> ((hi.lo)=w911:u16)
            n307 = Join Numbers(hi=w911, lo=w912) -> ((hi.lo)=w910:u32)
            "out_io1 2" <- w910
            n308 = Multiply(x=0.0201416015625, y=w910) -> (x*y=→"x*y":dbl)
          }
        }
        "CurrSp Graph" <- w789
        n309 = call "CheckStr.vi"("String"=w793) -> ("s? t:f"=w795:string)
        n310 = Concatenate Strings(w795, w799) -> (w797:string)
        "String 2" <- w797
      }
    }
  }
  n311 = while {
    tunnel: [TRUE] -> _
    tunnel: w29 -> [_]
    tunnel: w6 -> [w931]
    tunnel: [w930] -> _
    tunnel: errorcluster {"status"=FALSE, "code"=0, "source"=""} -> [w929]
    shift-right: [w928] -> _
    shift-left: refnum<visa-resource-name> refnum ("Value") -> [w925]
    shift-right: [w926] -> _
    shift-left: FALSE ("Value") -> [w924]
    shift-right: [w927] -> _
    shift-left: FALSE ("Plot_T") -> [w923]
    tunnel: ["Flag Stop R"] -> _
    stop <- "Flag Stop R" stop-if-true
    # "Receive Task"
    n312 = case shown="False" w923 {
      tunnel: [w937 w939] -> w933
      tunnel: [w934 w938] -> w926
      tunnel: w925 -> [_ w939]
      tunnel: w924 -> [_ w938]
      frame False {
        n313 = control-ref of="VISA"() -> (w936:refnum<vi>)
        n314 = control-ref of="CommIcon"() -> (w935:refnum<vi>)
        n315 = property class="Bool (strict)"(reference=w935) -> ("Value"=w934:bool)  [unwired: 1 in, 2 out]
        n316 = property class="VISAName"(reference=w936) -> ("Value"=w937:refnum<visa-resource-name>)  [unwired: 1 in, 2 out]
      }
      frame True {
      }
    }
    n317 = case shown="False" w926 {
      tunnel: w929 -> [w952 w997]
      tunnel: w933 -> [w949 w998]
      tunnel: [w941 w998] -> w928
      tunnel: [w953 w997] -> w930
      tunnel: w931 -> [w942 w996]
      tunnel: [w954 w996] -> _
      tunnel: [w951 FALSE ("Plot_T")] -> w927
      tunnel: w923 -> [w940 _]
      frame False {
        (unwired) u32 8 ("byte count")
        n318 = VISA Read(VISA resource name=w949, byte count=u32 1, error in (no error)=w952) -> (VISA resource name out=w944:refnum<visa-resource-name>, read buffer=w945:string, error out=w943:errorcluster)  [unwired: 1 out]
        n319 = String To Byte Array(string=w945) -> (unsigned byte array=w948:u8[])
        n320 = Index Array(array=w948, index=0) -> (element=w946:u8)
        n321 = case shown="75" w946 {
          tunnel: [w958 w976] -> w954
          tunnel: [w957 w975] -> w953
          tunnel: [FALSE w974] -> w951
          tunnel: w944 -> [w955 w970]
          tunnel: w943 -> [w957 w969]
          tunnel: w942 -> [w958 w962]
          tunnel: [w955 w961] -> w941
          tunnel: w940 -> [_ w960]
          frame 0, Default {
          }
          frame 75 {
            n322 = VISA Read(VISA resource name=w970, byte count=u32 3, error in (no error)=w969) -> (VISA resource name out=w965:refnum<visa-resource-name>, read buffer=w973:string, error out=w964:errorcluster)  [unwired: 1 out]
            n323 = String To Byte Array(string=w973) -> (unsigned byte array=w963:u8[])
            n324 = local read "Add Unit"() -> (w959:u8)
            n325 = Index Array(array=w963, index #1=0 ("index")) -> (element #1=w968:u8, element #2=w966:u8)  [unwired: 2 in, 1 out]
            n326 = Equal?(x=w959, y=w968) -> (x = y?=w967:bool)
            n327 = case shown="True" w967 {
              tunnel: [w980 w993] -> w976
              tunnel: [w978 w992] -> w975
              tunnel: [w977 w983] -> w974
              tunnel: w966 -> [_ w991]
              tunnel: w965 -> [w979 w990]
              tunnel: w964 -> [w978 w989]
              tunnel: w963 -> [_ w987]
              tunnel: w962 -> [w980 w984]
              tunnel: [w979 w982] -> w961
              tunnel: w960 -> [w977 w983]
              frame False {
              }
              frame True {
                n328 = VISA Read(VISA resource name=w990, byte count=w991, error in (no error)=w989) -> (VISA resource name out=w982:refnum<visa-resource-name>, read buffer=w981:string, error out=w988:errorcluster)  [unwired: 1 out]
                "RX" <- w981
                n329 = String To Byte Array(string=w981) -> (unsigned byte array=w986:u8[])
                n330 = Insert Into Array(array=w987, new element=w986) -> (w985:u8[])  [unwired: 1 in]
                n331 = Enqueue Element(queue=w984, element=w985, error in (no error)=w988) -> (queue out=w993:refnum<queue>, error out=w992:errorcluster)  [unwired: 2 out]
              }
            }
          }
        }
      }
      frame True {
        n332 = Wait (ms)(milliseconds to wait=u32 10) -> ()  [unwired: 1 out]
      }
    }
  }
  n333 = while {
    tunnel: w14 -> [_]
    tunnel: w13 -> [w1000]
    stop <- "Flag Stop T" stop-if-true
    # "Transmit task"
    n334 = control-ref of="VISA"() -> (w1004:refnum<vi>)
    n335 = control-ref of="CommIcon"() -> (w1005:refnum<vi>)
    n336 = property class="Bool (strict)"(reference=w1005) -> ("Value"=w999:bool)  [unwired: 1 in, 2 out]
    n337 = property class="VISAName"(reference=w1004) -> ("Value"=w1003:refnum<visa-resource-name>)  [unwired: 1 in, 2 out]
    n338 = case shown="False" w999 {
      tunnel: w1003 -> [w1007 _]
      tunnel: errorcluster {"status"=FALSE, "code"=0, "source"=""} -> [w1006 _]
      tunnel: w1000 -> [w1009 _]
      frame False {
        n339 = Get Queue Status(queue=w1009) -> (queue out=w1008:refnum<queue>, # elements in queue=w1010:i32)  [unwired: 1 in, 7 out]
        n340 = case shown="1, Default" w1010 {
          tunnel: w1008 -> [_ w1018]
          tunnel: w1007 -> [_ w1017]
          tunnel: w1006 -> [_ w1015]
          frame 0 {
            n341 = local write "TX"(FALSE ("TX")) -> ()
          }
          frame 1, Default {
            n342 = Dequeue Element(queue=w1018) -> (element=w1014:u8[])  [unwired: 1 in, 4 out]
            "Write array" <- w1014
            n343 = Byte Array To String(unsigned byte array=w1014) -> (string=w1012:string)
            "TX" <- w1012
            n344 = VISA Write(VISA resource name=w1017, write buffer=w1012, error in (no error)=w1015) -> (error out=→"err tx":errorcluster)  [unwired: 2 out]
            n345 = local write "TX"(TRUE ("TX")) -> ()
          }
        }
      }
      frame True {
        n346 = Wait (ms)(milliseconds to wait=u32 10) -> ()  [unwired: 1 out]
      }
    }
  }
